vi "BSON_bynary_bytes_to_i16_array.vi"(11 "BSONbytes":u8[](array[numeric])) -> (3 "i16_array":i16[](array[numeric]))   [LabVIEW 2015, in "BSON_convertors_Library.lvlib"]
uses:
  BSON_convertors_Library.lvlib
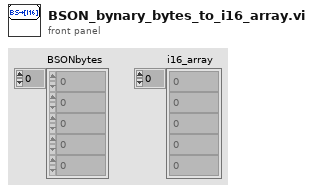
[diagram p1: front panel]
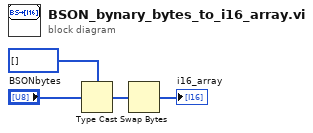
[diagram p0: block diagram]
diagram:
  n1 = Type Cast(type=i16[] [], x="BSONbytes") -> (*(type *) &x=w2:i16[])
  n2 = Swap Bytes(anything=w2) -> (byte swapped=→"i16_array":i16[])
